vi "Text To boolean.vi"(10 "eigen tekst":string, 11 "Numeric":i32) -> (2 "Letter":bool[][][](array[boolean]))   [LabVIEW 2013]
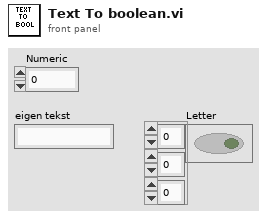
[diagram p1: front panel]
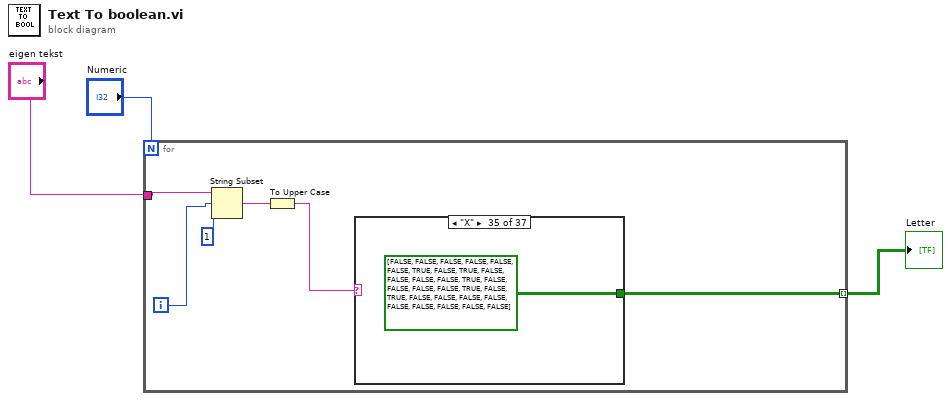
[diagram p0: block diagram]
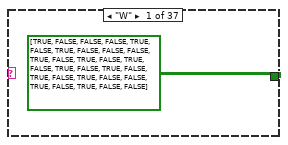
[diagram p2: hidden frame]
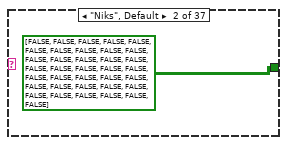
[diagram p3: hidden frame]
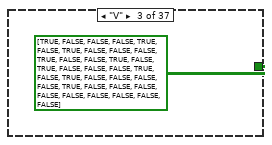
[diagram p4: hidden frame]
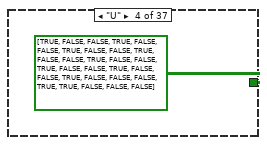
[diagram p5: hidden frame]
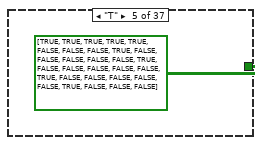
[diagram p6: hidden frame]
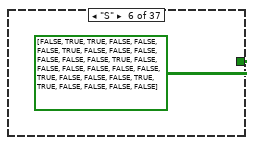
[diagram p7: hidden frame]
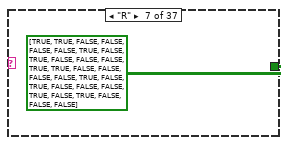
[diagram p8: hidden frame]
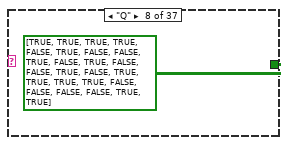
[diagram p9: hidden frame]
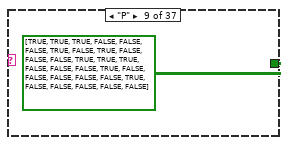
[diagram p10: hidden frame]
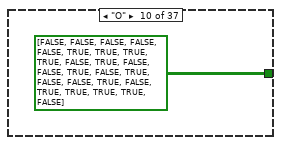
[diagram p11: hidden frame]
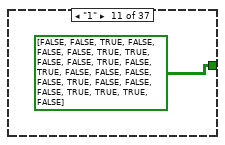
[diagram p12: hidden frame]
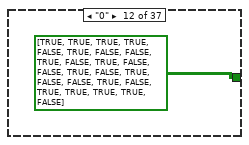
[diagram p13: hidden frame]
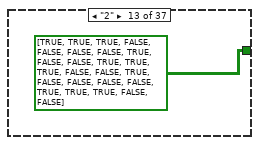
[diagram p14: hidden frame]
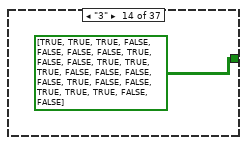
[diagram p15: hidden frame]
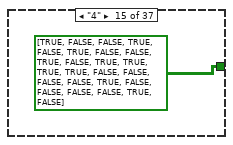
[diagram p16: hidden frame]
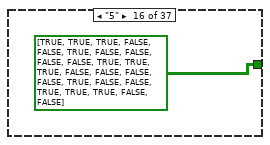
[diagram p17: hidden frame]
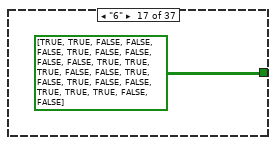
[diagram p18: hidden frame]
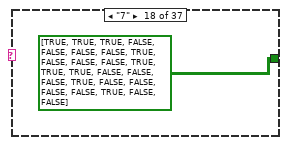
[diagram p19: hidden frame]
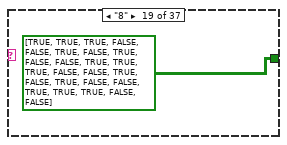
[diagram p20: hidden frame]
diagram:
  n1 = for {
    N: "Numeric" -> [_]
    tunnel: "eigen tekst" -> [w9]
    tunnel: [w4] -> w2 mode=indexing
    i -> [w8]
    n2 = String Subset(string=w9, offset (0)=w8, length (rest)=1 ("length (rest)")) -> (substring=w6:string)
    n3 = To Upper Case(1:w6) -> (0:w5:string)
    n4 = case shown="\"X\"" w5 {
      tunnel: [bool[][] [[TRUE, FALSE, FALSE, FALSE, TRUE, FALSE], [TRUE, FALSE, FALSE, FALSE, TRUE, FALSE], [TRUE, FALSE, TRUE, FALSE, TRUE, FALSE], [TRUE, FALSE, TRUE, FALSE, TRUE, FALSE], [FALSE, TRUE, FALSE, TRUE, FALSE, FALSE]] ("Letter") bool[][] [[FALSE, FALSE, FALSE, FALSE, FALSE, FALSE], [FALSE, FALSE, FALSE, FALSE, FALSE, FALSE], [FALSE, FALSE, FALSE, FALSE, FALSE, FALSE], [FALSE, FALSE, FALSE, FALSE, FALSE, FALSE], [FALSE, FALSE, FALSE, FALSE, FALSE, FALSE], [FALSE, FALSE, FALSE, FALSE, FALSE, FALSE]] ("Letter") bool[][] [[TRUE, FALSE, FALSE, FALSE, TRUE, FALSE], [TRUE, FALSE, FALSE, FALSE, TRUE, FALSE], [FALSE, TRUE, FALSE, TRUE, FALSE, FALSE], [FALSE, TRUE, FALSE, TRUE, FALSE, FALSE], [FALSE, FALSE, TRUE, FALSE, FALSE, FALSE], [FALSE, FALSE, FALSE, FALSE, FALSE, FALSE]] ("Letter") bool[][] [[TRUE, FALSE, FALSE, TRUE, FALSE, FALSE], [TRUE, FALSE, FALSE, TRUE, FALSE, FALSE], [TRUE, FALSE, FALSE, TRUE, FALSE, FALSE], [TRUE, FALSE, FALSE, TRUE, FALSE, FALSE], [FALSE, TRUE, TRUE, FALSE, FALSE, FALSE]] ("Letter") bool[][] [[TRUE, TRUE, TRUE, TRUE, TRUE, FALSE], [FALSE, FALSE, TRUE, FALSE, FALSE, FALSE], [FALSE, FALSE, TRUE, FALSE, FALSE, FALSE], [FALSE, FALSE, TRUE, FALSE, FALSE, FALSE], [FALSE, FALSE, TRUE, FALSE, FALSE, FALSE]] ("Letter") bool[][] [[FALSE, TRUE, TRUE, FALSE, FALSE, FALSE], [TRUE, FALSE, FALSE, FALSE, FALSE, FALSE], [FALSE, TRUE, FALSE, FALSE, FALSE, FALSE], [FALSE, FALSE, TRUE, FALSE, FALSE, FALSE], [TRUE, TRUE, FALSE, FALSE, FALSE, FALSE]] ("Letter") bool[][] [[TRUE, TRUE, FALSE, FALSE, FALSE, FALSE], [TRUE, FALSE, TRUE, FALSE, FALSE, FALSE], [TRUE, TRUE, FALSE, FALSE, FALSE, FALSE], [TRUE, FALSE, TRUE, FALSE, FALSE, FALSE], [TRUE, FALSE, TRUE, FALSE, FALSE, FALSE]] ("Letter") bool[][] [[TRUE, TRUE, TRUE, TRUE, FALSE], [TRUE, FALSE, FALSE, TRUE, FALSE], [TRUE, FALSE, FALSE, TRUE, FALSE], [TRUE, TRUE, TRUE, TRUE, FALSE], [FALSE, FALSE, FALSE, TRUE, TRUE]] ("Letter") bool[][] [[TRUE, TRUE, TRUE, FALSE, FALSE, FALSE], [TRUE, FALSE, TRUE, FALSE, FALSE, FALSE], [TRUE, TRUE, TRUE, FALSE, FALSE, FALSE], [TRUE, FALSE, FALSE, FALSE, FALSE, FALSE], [TRUE, FALSE, FALSE, FALSE, FALSE, FALSE]] ("Letter") bool[][] [[FALSE, FALSE, FALSE, FALSE, FALSE], [TRUE, TRUE, TRUE, TRUE, FALSE], [TRUE, FALSE, FALSE, TRUE, FALSE], [TRUE, FALSE, FALSE, TRUE, FALSE], [TRUE, TRUE, TRUE, TRUE, FALSE]] ("Letter") bool[][] [[FALSE, FALSE, TRUE, FALSE, FALSE], [FALSE, TRUE, TRUE, FALSE, FALSE], [TRUE, FALSE, TRUE, FALSE, FALSE], [FALSE, FALSE, TRUE, FALSE, FALSE], [FALSE, TRUE, TRUE, TRUE, FALSE]] ("Letter") bool[][] [[TRUE, TRUE, TRUE, TRUE, FALSE], [TRUE, FALSE, FALSE, TRUE, FALSE], [TRUE, FALSE, FALSE, TRUE, FALSE], [TRUE, FALSE, FALSE, TRUE, FALSE], [TRUE, TRUE, TRUE, TRUE, FALSE]] ("Letter") bool[][] [[TRUE, TRUE, TRUE, FALSE, FALSE], [FALSE, FALSE, TRUE, FALSE, FALSE], [TRUE, TRUE, TRUE, FALSE, FALSE], [TRUE, FALSE, FALSE, FALSE, FALSE], [TRUE, TRUE, TRUE, FALSE, FALSE]] ("Letter") bool[][] [[TRUE, TRUE, TRUE, FALSE, FALSE], [FALSE, FALSE, TRUE, FALSE, FALSE], [TRUE, TRUE, TRUE, FALSE, FALSE], [FALSE, FALSE, TRUE, FALSE, FALSE], [TRUE, TRUE, TRUE, FALSE, FALSE]] ("Letter") bool[][] [[TRUE, FALSE, FALSE, TRUE, FALSE], [TRUE, FALSE, FALSE, TRUE, FALSE], [TRUE, TRUE, TRUE, TRUE, FALSE], [FALSE, FALSE, FALSE, TRUE, FALSE], [FALSE, FALSE, FALSE, TRUE, FALSE]] ("Letter") bool[][] [[TRUE, TRUE, TRUE, FALSE, FALSE], [TRUE, FALSE, FALSE, FALSE, FALSE], [TRUE, TRUE, TRUE, FALSE, FALSE], [FALSE, FALSE, TRUE, FALSE, FALSE], [TRUE, TRUE, TRUE, FALSE, FALSE]] ("Letter") bool[][] [[TRUE, TRUE, FALSE, FALSE, FALSE], [TRUE, FALSE, FALSE, FALSE, FALSE], [TRUE, TRUE, TRUE, FALSE, FALSE], [TRUE, FALSE, TRUE, FALSE, FALSE], [TRUE, TRUE, TRUE, FALSE, FALSE]] ("Letter") bool[][] [[TRUE, TRUE, TRUE, FALSE, FALSE], [FALSE, FALSE, TRUE, FALSE, FALSE], [FALSE, TRUE, TRUE, TRUE, FALSE], [FALSE, FALSE, TRUE, FALSE, FALSE], [FALSE, FALSE, TRUE, FALSE, FALSE]] ("Letter") bool[][] [[TRUE, TRUE, TRUE, FALSE, FALSE], [TRUE, FALSE, TRUE, FALSE, FALSE], [TRUE, TRUE, TRUE, FALSE, FALSE], [TRUE, FALSE, TRUE, FALSE, FALSE], [TRUE, TRUE, TRUE, FALSE, FALSE]] ("Letter") bool[][] [[TRUE, TRUE, TRUE, FALSE, FALSE], [TRUE, FALSE, TRUE, FALSE, FALSE], [TRUE, TRUE, TRUE, FALSE, FALSE], [FALSE, FALSE, TRUE, FALSE, FALSE], [TRUE, TRUE, TRUE, FALSE, FALSE]] ("Letter") bool[][] [[TRUE, FALSE, FALSE, TRUE, FALSE], [TRUE, TRUE, FALSE, TRUE, FALSE], [TRUE, FALSE, TRUE, TRUE, FALSE], [TRUE, FALSE, FALSE, TRUE, FALSE], [TRUE, FALSE, FALSE, TRUE, FALSE]] ("Letter") bool[][] [[TRUE, FALSE, FALSE, FALSE, TRUE, FALSE], [TRUE, TRUE, FALSE, TRUE, TRUE, FALSE], [TRUE, FALSE, TRUE, FALSE, TRUE, FALSE], [TRUE, FALSE, FALSE, FALSE, TRUE, FALSE], [TRUE, FALSE, FALSE, FALSE, TRUE, FALSE]] ("Letter") bool[][] [[TRUE, FALSE, FALSE, FALSE, FALSE, FALSE], [TRUE, FALSE, FALSE, FALSE, FALSE, FALSE], [TRUE, FALSE, FALSE, FALSE, FALSE, FALSE], [TRUE, FALSE, FALSE, FALSE, FALSE, FALSE], [TRUE, TRUE, TRUE, TRUE, FALSE, FALSE]] ("Letter") bool[][] [[TRUE, FALSE, FALSE, TRUE, FALSE], [TRUE, FALSE, TRUE, FALSE, FALSE], [TRUE, TRUE, FALSE, FALSE, FALSE], [TRUE, FALSE, TRUE, FALSE, FALSE], [TRUE, FALSE, FALSE, TRUE, FALSE]] ("Letter") bool[][] [[FALSE, FALSE, TRUE, FALSE, FALSE], [FALSE, FALSE, TRUE, FALSE, FALSE], [FALSE, FALSE, TRUE, FALSE, FALSE], [FALSE, FALSE, TRUE, FALSE, FALSE], [TRUE, TRUE, FALSE, FALSE, FALSE]] ("Letter") bool[][] [[FALSE, TRUE, TRUE, TRUE, FALSE], [FALSE, FALSE, TRUE, FALSE, FALSE], [FALSE, FALSE, TRUE, FALSE, FALSE], [FALSE, FALSE, TRUE, FALSE, FALSE], [FALSE, TRUE, TRUE, TRUE, FALSE]] ("Letter") bool[][] [[TRUE, FALSE, FALSE, TRUE, FALSE], [TRUE, FALSE, FALSE, TRUE, FALSE], [TRUE, TRUE, TRUE, TRUE, FALSE], [TRUE, FALSE, FALSE, TRUE, FALSE], [TRUE, FALSE, FALSE, TRUE, FALSE]] ("Letter") bool[][] [[TRUE, TRUE, TRUE, TRUE, FALSE, FALSE], [TRUE, FALSE, FALSE, FALSE, FALSE, FALSE], [TRUE, FALSE, TRUE, TRUE, FALSE, FALSE], [TRUE, FALSE, FALSE, TRUE, FALSE, FALSE], [TRUE, TRUE, TRUE, TRUE, FALSE, FALSE]] ("Letter") bool[][] [[TRUE, TRUE, TRUE, FALSE, FALSE, FALSE], [TRUE, FALSE, FALSE, FALSE, FALSE, FALSE], [TRUE, TRUE, TRUE, FALSE, FALSE, FALSE], [TRUE, FALSE, FALSE, FALSE, FALSE, FALSE], [TRUE, FALSE, FALSE, FALSE, FALSE, FALSE]] ("Letter") bool[][] [[TRUE, TRUE, TRUE, FALSE, FALSE], [TRUE, FALSE, FALSE, FALSE, FALSE], [TRUE, TRUE, TRUE, FALSE, FALSE], [TRUE, FALSE, FALSE, FALSE, FALSE], [TRUE, TRUE, TRUE, FALSE, FALSE]] ("Letter") bool[][] [[TRUE, TRUE, FALSE, FALSE, FALSE], [TRUE, FALSE, TRUE, FALSE, FALSE], [TRUE, FALSE, TRUE, FALSE, FALSE], [TRUE, FALSE, TRUE, FALSE, FALSE], [TRUE, TRUE, FALSE, FALSE, FALSE]] ("Letter") bool[][] [[TRUE, TRUE, TRUE, FALSE, FALSE], [TRUE, FALSE, FALSE, FALSE, FALSE], [TRUE, FALSE, FALSE, FALSE, FALSE], [TRUE, FALSE, FALSE, FALSE, FALSE], [TRUE, TRUE, TRUE, FALSE, FALSE]] ("Letter") bool[][] [[TRUE, TRUE, FALSE, FALSE, FALSE], [TRUE, FALSE, TRUE, FALSE, FALSE], [TRUE, TRUE, FALSE, FALSE, FALSE], [TRUE, FALSE, TRUE, FALSE, FALSE], [TRUE, TRUE, FALSE, FALSE, FALSE]] ("Letter") bool[][] [[FALSE, TRUE, TRUE, FALSE, FALSE], [TRUE, FALSE, FALSE, TRUE, FALSE], [TRUE, TRUE, TRUE, TRUE, FALSE], [TRUE, FALSE, FALSE, TRUE, FALSE], [TRUE, FALSE, FALSE, TRUE, FALSE]] ("Letter") bool[][] [[FALSE, FALSE, FALSE, FALSE, FALSE, FALSE], [TRUE, FALSE, TRUE, FALSE, FALSE, FALSE], [FALSE, TRUE, FALSE, FALSE, FALSE, FALSE], [TRUE, FALSE, TRUE, FALSE, FALSE, FALSE], [FALSE, FALSE, FALSE, FALSE, FALSE, FALSE]] ("Letter") bool[][] [[TRUE, FALSE, FALSE, FALSE, TRUE, FALSE], [FALSE, TRUE, FALSE, TRUE, FALSE, FALSE], [FALSE, FALSE, TRUE, FALSE, FALSE, FALSE], [FALSE, FALSE, TRUE, FALSE, FALSE, FALSE], [FALSE, FALSE, TRUE, FALSE, FALSE, FALSE]] ("Letter") bool[][] [[FALSE, TRUE, TRUE, TRUE, TRUE], [FALSE, FALSE, FALSE, TRUE, FALSE], [FALSE, FALSE, TRUE, FALSE, FALSE], [FALSE, TRUE, FALSE, FALSE, FALSE], [FALSE, TRUE, TRUE, TRUE, TRUE]] ("Letter")] -> w4
      frame "W" {
      }
      frame "Niks", Default {
      }
      frame "V" {
      }
      frame "U" {
      }
      frame "T" {
      }
      frame "S" {
      }
      frame "R" {
      }
      frame "Q" {
      }
      frame "P" {
      }
      frame "O" {
      }
      frame "1" {
      }
      frame "0" {
      }
      frame "2" {
      }
      frame "3" {
      }
      frame "4" {
      }
      frame "5" {
      }
      frame "6" {
      }
      frame "7" {
      }
      frame "8" {
      }
      frame "9" {
      }
      frame "N" {
      }
      frame "M" {
      }
      frame "L" {
      }
      frame "K" {
      }
      frame "J" {
      }
      frame "I" {
      }
      frame "H" {
      }
      frame "G" {
      }
      frame "F" {
      }
      frame "E" {
      }
      frame "D" {
      }
      frame "C" {
      }
      frame "B" {
      }
      frame "A" {
      }
      frame "X" {
      }
      frame "Y" {
      }
      frame "Z" {
      }
    }
  }
  "Letter" <- w2
